vi "Apply_17V_to_VBAT.vi"(3 "error in":errorcluster) -> (10 "error out":errorcluster)   [LabVIEW 2015]
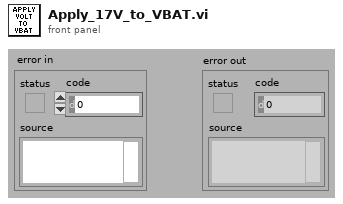
[diagram p1: front panel]
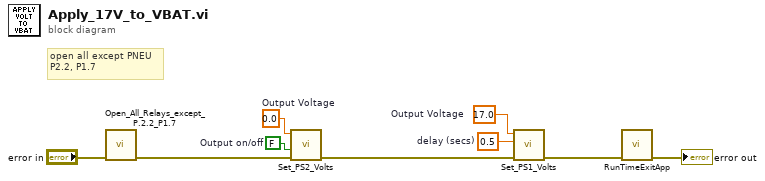
[diagram p0: block diagram]
diagram:
  w1 = 0.0  # Output Voltage
  w5 = FALSE  # Output on/off
  w6 = 0.5  # delay (secs)
  w7 = 17.0  # Output Voltage
  # "open all except PNEU\nP2.2, P1.7"
  n1 = call "Open_All_Relays_except_P.2.2_P1.7.vi"("error in"="error in") -> ("error out"=w3:errorcluster)  [unwired: 8 in]
  n2 = call "Set_PS2_Volts.vi"("error in"=w3, "Output on/off"=w5, "Output Voltage"=w1) -> ("error out"=w2:errorcluster)  [unwired: 6 in, 2 out]
  n3 = call "Set_PS1_Volts.vi"("error in"=w2, "delay (secs)"=w6, "Output Voltage"=w7) -> ("error out"=w4:errorcluster)  [unwired: 6 in, 2 out]
  n4 = call "RunTimeExitApp.vi"("error in (no error)"=w4) -> ("error out"=→"error out":errorcluster)  [unwired: 10 in]
